vi "Search Complex Pair with Approximation.vi"(10 "tolerance for complex pair":dbl=1e-10, 11 "Complex Numbers":cdb[](array[numeric])) -> (2 "Complex Pair Numbers":cdb[](array[numeric]), 3 "Pure Complex Numbers":cdb[](array[numeric]))   [LabVIEW 2020, in "NI_AALPro.lvlib"]
uses:
  NI_AALPro.lvlib
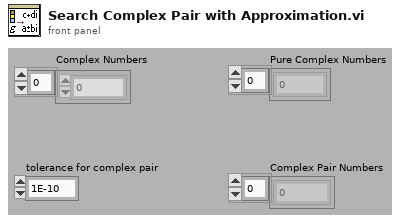
[diagram p1: front panel]
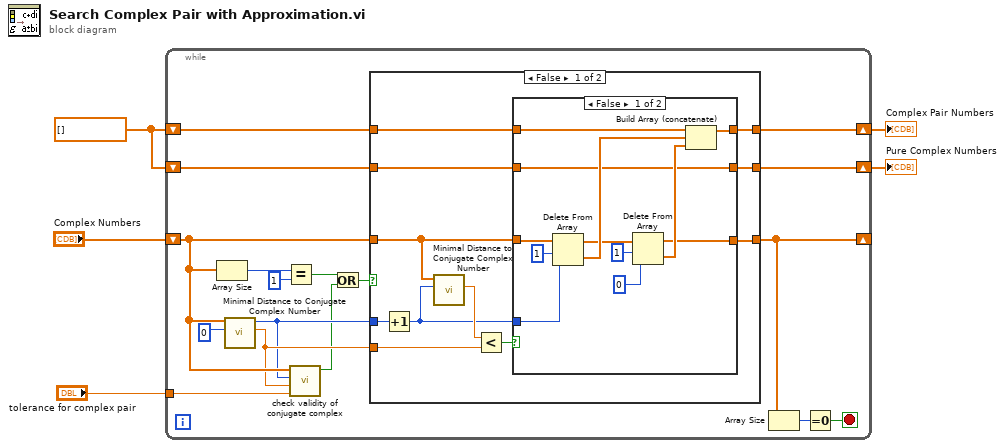
[diagram p0: block diagram]
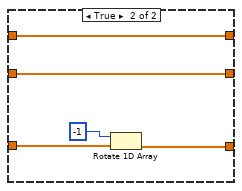
[diagram p2: hidden frame]
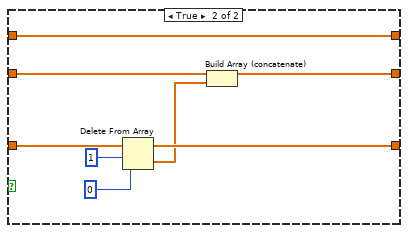
[diagram p3: hidden frame]
diagram:
  w2 = cdb[] [] ("CDB")
  n1 = while {
    tunnel: "tolerance for complex pair" -> [w6]
    shift-right: [w16] -> w1
    shift-left: w2 -> [w17]
    shift-right: [w22] -> w3
    shift-left: w2 -> [w18]
    shift-right: [w21] -> _
    shift-left: "Complex Numbers" -> [w10]
    stop <- w19 stop-if-true
    n2 = Array Size(array=w10) -> (size(s)=w15:i32)
    n3 = call "Minimal Distance to Conjugate Complex Number.vi"("index"=0, "Complex Number Array"=w10) -> ("min distance to (z)*"=w9:dbl, "min distance index"=w8:i32)  [unwired: 8 in]
    n4 = Equal?(x=w15, y=1) -> (x = y?=w13:bool)
    n5 = call "check validity of conjugate complex.vi"("tolerance for complex pair"=w6, "min distance to (z)*"=w9, "min distance index"=w8, "Complex Numbers"=w10) -> ("out of tolerance?"=w7:bool)  [unwired: 7 in]
    n6 = Or(x=w13, y=w7) -> (x .or. y?=w12:bool)
    n7 = case shown="False" w12 {
      tunnel: w8 -> [w33 _]
      tunnel: w10 -> [w23 w58]
      tunnel: [w26 w55] -> w21
      tunnel: [w28 w51] -> w22
      tunnel: w9 -> [w32 _]
      tunnel: w18 -> [w29 w53]
      tunnel: w17 -> [w30 w54]
      tunnel: [w27 w54] -> w16
      frame False {
        n8 = Increment(x=w33) -> (x+1=w24:i32)
        n9 = call "Minimal Distance to Conjugate Complex Number.vi"("index"=w24, "Complex Number Array"=w23) -> ("min distance to (z)*"=w25:dbl)  [unwired: 8 in, 1 out]
        n10 = Less?(x=w25, y=w32) -> (x < y?=w31:bool)
        n11 = case shown="False" w31 {
          tunnel: w24 -> [w43 _]
          tunnel: w23 -> [w45 w48]
          tunnel: w30 -> [w42 w50]
          tunnel: w29 -> [w34 w49]
          tunnel: [w34 w49] -> w28
          tunnel: [w36 w50] -> w27
          tunnel: [w35 w47] -> w26
          frame False {
            n12 = Delete From Array(array=w45, length=1, index=w43) -> (deleted portion=w41:cdb[], array with subset deleted=w40:cdb[])
            n13 = Delete From Array(array=w40, length=1, index=0) -> (deleted portion=w37:cdb[], array with subset deleted=w35:cdb[])
            n14 = Build Array (concatenate)(w42, w41, w37) -> (w36:cdb[])
          }
          frame True {
            n15 = Rotate 1D Array(1:w48, 2:-1 ("n")) -> (0:w47:cdb[])
          }
        }
      }
      frame True {
        n16 = Delete From Array(array=w58, length=1, index=0) -> (deleted portion=w52:cdb[], array with subset deleted=w55:cdb[])
        n17 = Build Array (concatenate)(w53, w52) -> (w51:cdb[])
      }
    }
    n18 = Array Size(array=w21) -> (size(s)=w20:i32)
    n19 = Equal To 0?(x=w20) -> (x = 0?=w19:bool)
  }
  "Pure Complex Numbers" <- w3
  "Complex Pair Numbers" <- w1
